vi "Line or Circle move.vi"(8 "motion":T2, 9 "draw point Cluster":T3, 10 "new/data speed":bool, 11 "Motion.lvclass":refnum<class "Motion.lvclass">) -> (3 "Motion.lvclass 2":refnum<class "Motion.lvclass">)   [LabVIEW 2016]
uses:
  Classes/Controller/Motion/Motion Folder/Motion.lvclass
  Classes/Controller/Motion/A3200 Folder/A3200.lvclass
  Classes/Controller/Dispenser/Ultimus V2 Folder/Ultimus V2.lvclass
  Classes/Controller/I-O/NI-DAQ Folder/NI-DAQ.lvclass
  Classes/Controller/I-O/I-O Folder/I-O.lvclass
  Classes/Controller/Dispenser/Dispenser Folder/Dispenser.lvclass
panel:
  out "controller out":T1
  in  "controller in":T1
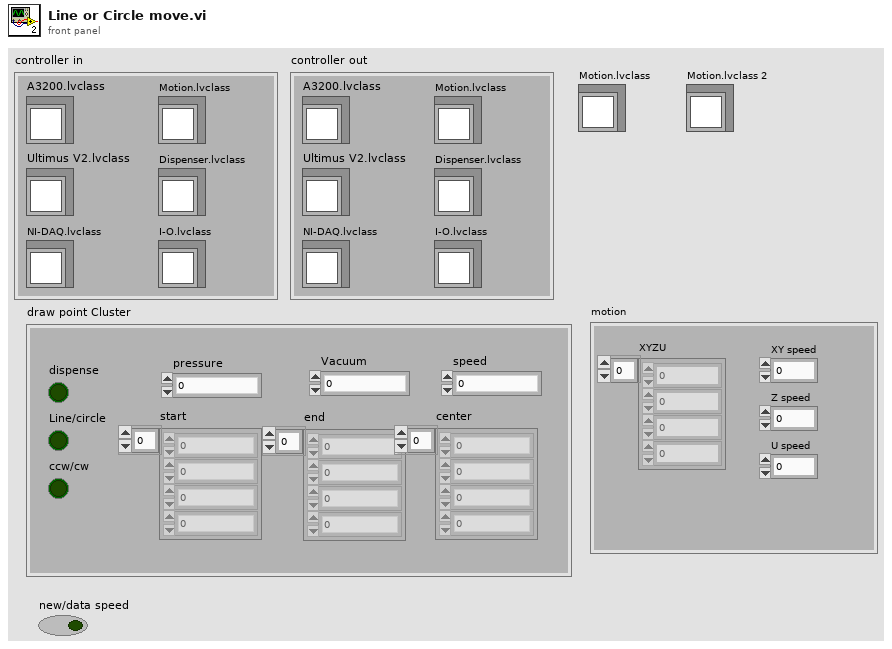
[diagram p1: front panel]
types:
  T1 = cluster{"A3200.lvclass":refnum<class "A3200.lvclass">, "Ultimus V2.lvclass":refnum<class "Ultimus V2.lvclass">, "NI-DAQ.lvclass":refnum<class "NI-DAQ.lvclass">, "Motion.lvclass":refnum<class "Motion.lvclass">, "I-O.lvclass":refnum<class "I-O.lvclass">, "Dispenser.lvclass":refnum<class "Dispenser.lvclass">}
  T2 = cluster{"XYZU ":dbl[], "XY speed":dbl, "Z speed":dbl, "U speed":dbl}
  T3 = cluster{"dispense":bool, "Line/circle":bool, "ccw/cw":bool, "pressure":dbl, "speed":dbl, "start":dbl[], "end":dbl[], "center":dbl[], "Vacuum":dbl}
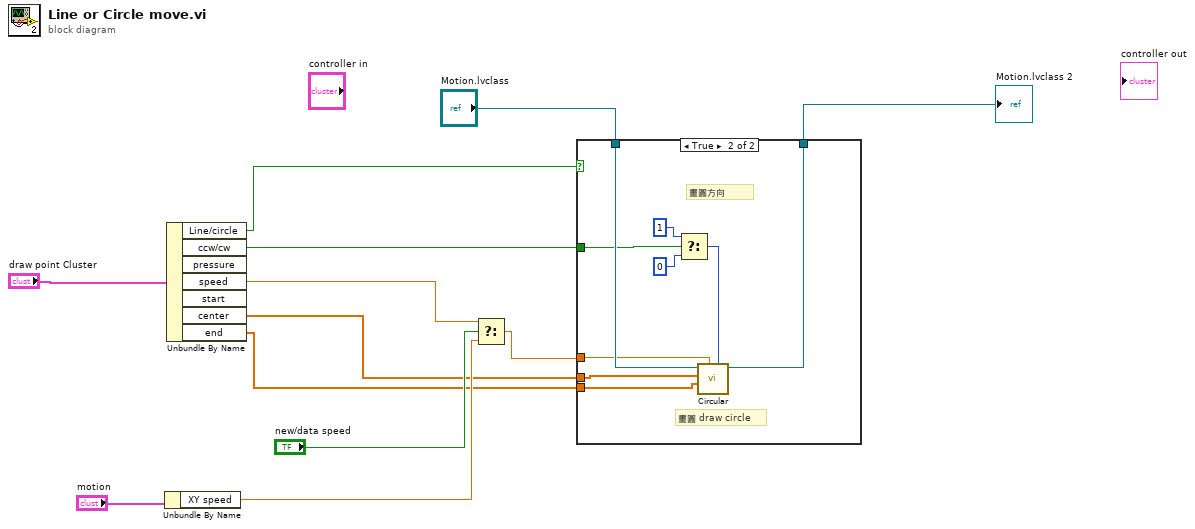
[diagram p0: block diagram]
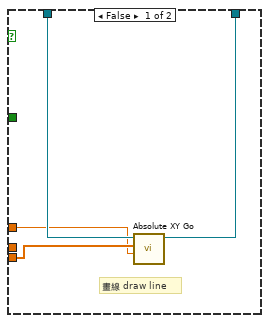
[diagram p2: hidden frame]
diagram:
  n1 = Unbundle By Name("motion") -> ("XY speed"=w8:dbl)
  n2 = Unbundle By Name("draw point Cluster") -> ("Line/circle"=w6:bool, "ccw/cw"=w5:bool, "speed"=w7:dbl, "center"=w3:dbl[], "end"=w4:dbl[])  [unwired: 2 out]
  n3 = Select(t=w7, s="new/data speed", f=w8) -> (s? t:f=w11:dbl)
  n4 = case shown="True" w6 {
    tunnel: "Motion.lvclass" -> [w16 w25]
    tunnel: [w15 w24] -> w1
    tunnel: w11 -> [w13 w20]
    tunnel: w5 -> [_ w19]
    tunnel: w3 -> [_ w18]
    tunnel: w4 -> [w14 w17]
    frame False {
      # "畫線 draw line"
      n5 = call-dynamic "Absolute XY Go.vi"("Speed"=w13, "XY"=w14, "Motion in"=w16) -> ("Motion out"=w15:refnum<class "Motion.lvclass">)  [unwired: 7 in, 1 out]
    }
    frame True {
      # "畫圓方向"
      # "畫圓 draw circle"
      n6 = Select(t=1, s=w19, f=0) -> (s? t:f=w23:i32)
      n7 = call-dynamic "Circular.vi"("Direction"=w23, "Speed"=w20, "XY End"=w17, "XY Center"=w18, "Motion in"=w25) -> ("Motion out"=w24:refnum<class "Motion.lvclass">)  [unwired: 5 in, 1 out]
    }
  }
  "Motion.lvclass 2" <- w1
